vi "HVSCommunication.vi"(8 "error in (no error)":errorcluster, 11 "VISA in":refnum<visa-resource-name>) -> (0 "error out":errorcluster, 2 "HVS Data Array":dbl[](array[numeric]), 3 "VISA out":refnum<visa-resource-name>)   [LabVIEW 2013]
doc: "Use this template to build a VI to use as a subVI."
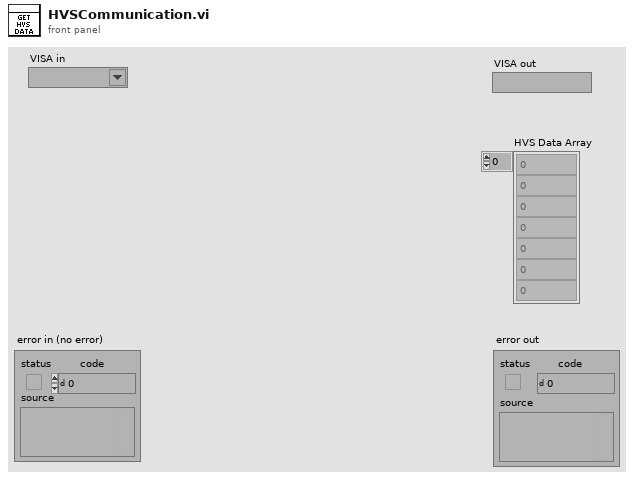
[diagram p1: front panel]
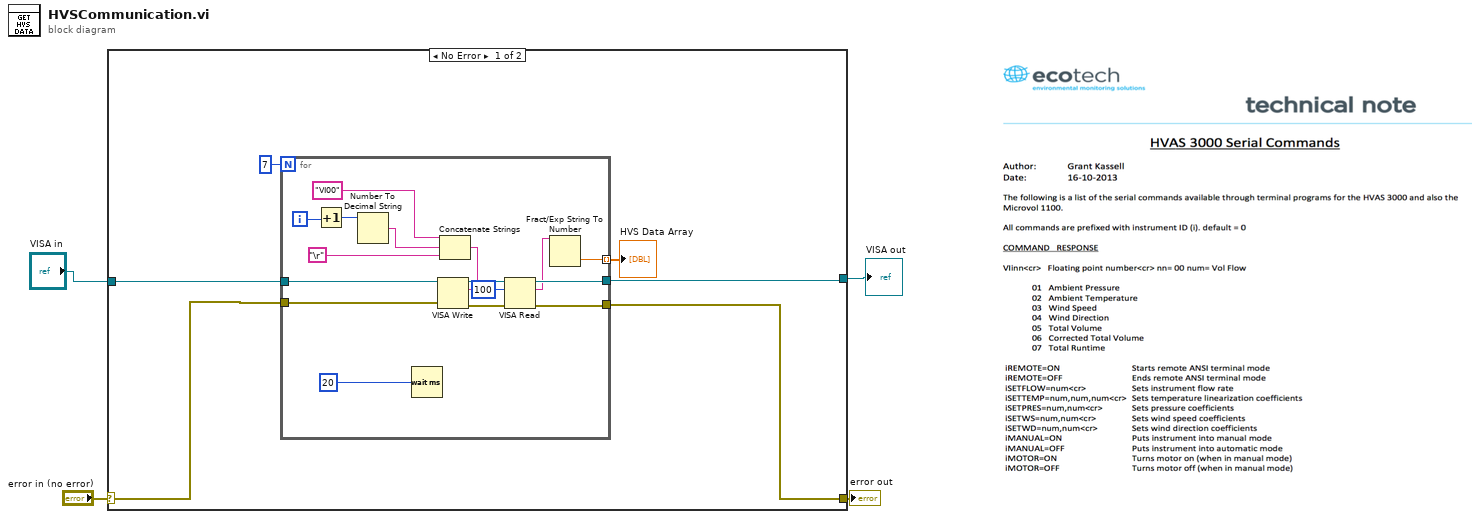
[diagram p0: block diagram]
diagram:
  n1 = case shown="No Error" "error in (no error)" {
    selector: "error in (no error)" -> [w7 w28]
    tunnel: [w8 w28] -> w3
    tunnel: "VISA in" -> [w6 w27]
    tunnel: [w5 w27] -> w1
    frame No Error {
      n2 = for {
        N: 7 -> [_]
        tunnel: w7 -> [w26]
        tunnel: [w21] -> w8
        tunnel: [w20] -> w5
        tunnel: [w12] -> w9 mode=indexing
        tunnel: w6 -> [w11]
        i -> [w16]
        n3 = Increment(x=w16) -> (x+1=w14:i32)
        n4 = Number To Decimal String(number=w14) -> (decimal integer string=w13:string)  [unwired: 1 in]
        n5 = Wait (ms)(milliseconds to wait=u32 20) -> ()  [unwired: 1 out]
        n6 = Concatenate Strings("VI00" ("write buffer"), w13, "\r") -> (w24:string)
        n7 = VISA Write(VISA resource name=w11, write buffer=w24, error in (no error)=w26) -> (VISA resource name out=w22:refnum<visa-resource-name>, error out=w23:errorcluster)  [unwired: 1 out]
        n8 = VISA Read(VISA resource name=w22, byte count=u32 100, error in (no error)=w23) -> (VISA resource name out=w20:refnum<visa-resource-name>, read buffer=w18:string, error out=w21:errorcluster)  [unwired: 1 out]
        n9 = Fract/Exp String To Number(string=w18) -> (number=w12:dbl)  [unwired: 3 in, 1 out]
      }
      "HVS Data Array" <- w9
    }
    frame Error {
    }
  }
  "error out" <- w3
  "VISA out" <- w1
